vi "pointandarrow.vi"(8 "alpha":dbl[](array[numeric]), 9 "u":dbl[](array[numeric]), 10 "index":i32, 11 "picture":picture) -> (3 "new picture":picture)   [LabVIEW 2014]
uses:
  <vilib>/imath/engines/lvmath2/RunTimeEngine/NodeEndStatement/NIMS_NodeEndStatement_Output.vi
  <instcachedir>/0/NIMS_NodeEndStatement_Output_53EC0D466D134D7ABD903AC30B43404B.lvgen/NIMS_NodeEndStatement_Output_53EC0D466D134D7ABD903AC30B43404B_001.vi
  <vilib>/imath/engines/lvmath2/RunTimeEngine/ErrorHandling/NIMS_Finalize Error.vi
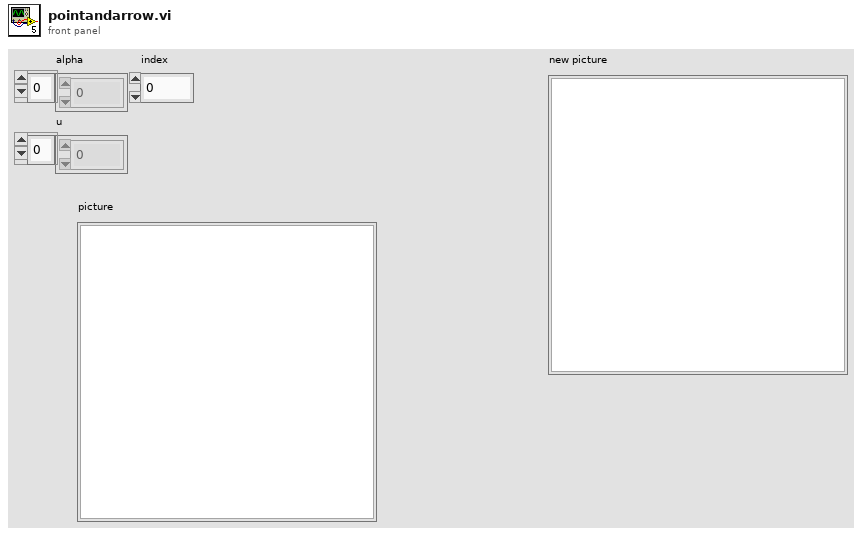
[diagram p1: front panel]
types:
  T1 = cluster{"Width":u16, "Style":enum32{"Solid", "Dash", "Dot", "DashDot", "DashDotDot"}}
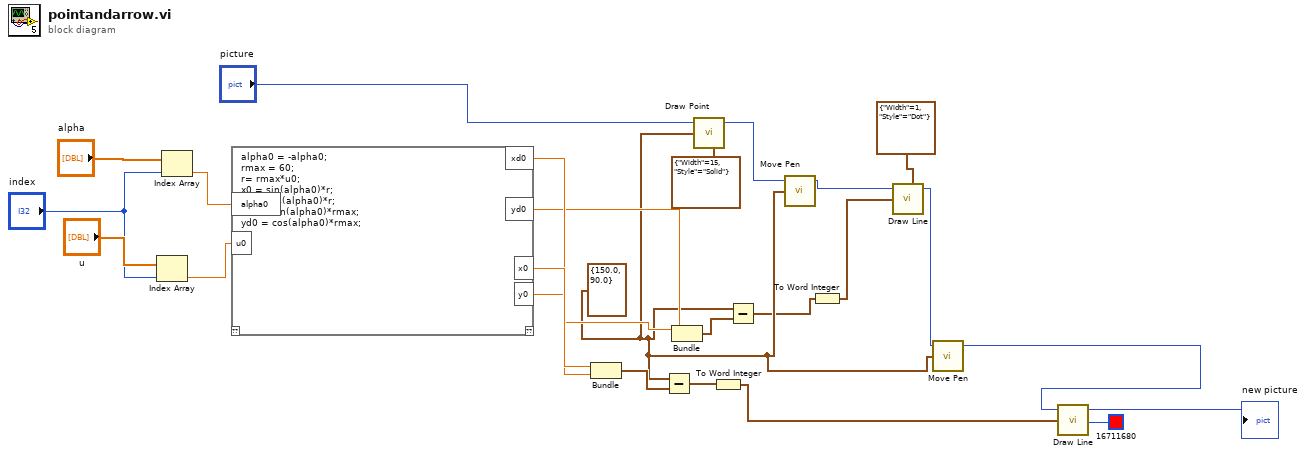
[diagram p0: block diagram]
diagram:
  w10 = cluster{dbl, dbl} {150.0, 90.0} ("new position")
  n1 = Index Array(array="u", index="index") -> (element=w4:dbl)
  n2 = Index Array(array="alpha", index="index") -> (element=w7:dbl)
  n3 = mathscript code="alpha0 = -alpha0;\nrmax = 60;\nr= rmax*u0;\nx0 = sin(alpha0)*r;\ny0 = cos(alpha0)*r;\nxd0 = sin(alpha0)*rmax;\nyd0 = cos(alpha0)*rmax;"("alpha0"=w7, "u0"=w4) -> ("x0"=w23:dbl, "y0"=w22:dbl, "xd0"=w12:dbl, "yd0"=w11:dbl)  [unwired: 1 in, 1 out]
  n4 = Bundle("x0"=w23, "y0"=w22) -> (w24:cluster{"x0":dbl, "y0":dbl})  [unwired: 1 in]
  n5 = Subtract(x=w10, y=w24) -> (x-y=w25:cluster{dbl, dbl})
  n6 = Bundle("xd0"=w12, "yd0"=w11) -> (w13:cluster{"xd0":dbl, "yd0":dbl})  [unwired: 1 in]
  n7 = call <vilib>:"Draw Point.vi"("picture"="picture", "point(x,y)"=w10, "pen"=T1 {"Width"=15, "Style"=enum."Solid"}) -> ("new picture"=w20:picture)  [unwired: 6 in]
  n8 = To Word Integer(number=w25) -> (16bit integer=w17:cluster{i16, i16})
  n9 = Subtract(x=w10, y=w13) -> (x-y=w9:cluster{dbl, dbl})
  n10 = call <vilib>:"Move Pen.vi"("new position"=w10, "picture"=w20) -> ("new picture"=w18:picture)  [unwired: 3 in]
  n11 = To Word Integer(number=w9) -> (16bit integer=w8:cluster{i16, i16})
  n12 = call <vilib>:"Draw Line.vi"("picture"=w18, "end point"=w8, "pen"=T1 {"Width"=1, "Style"=enum."Dot"}) -> ("new picture"=w15:picture)  [unwired: 6 in]
  n13 = call <vilib>:"Move Pen.vi"("new position"=w10, "picture"=w15) -> ("new picture"=w14:picture)  [unwired: 3 in]
  n14 = call <vilib>:"Draw Line.vi"("picture"=w14, "end point"=w17, "color(black)"=u32 16711680) -> ("new picture"=→"new picture":picture)  [unwired: 6 in]
